vi "HumanDashRead.vi"() -> (1 "DriveMode":T1, 2 "SlowMode":bool, 3 "FieldOriented":bool)   [LabVIEW 2023]
doc: "Human Network\n\nInput\n --Error in \n\nOutput\n --Error out"
uses:
  HumanGlobal.vi
  <vilib>/Rock Robotics/Network Tables/NT Read Boolean.vi
  <vilib>/Rock Robotics/Network Tables/NT Read Number.vi
  HumanDriveModeENUM.ctl
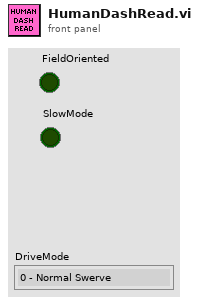
[diagram p1: front panel]
types:
  T1 = typedef "HumanDriveModeENUM.ctl" = enum16{"0 - Normal Swerve", "1 - Auto traj  - Left Speaker", "2 - Auto traj - Center Speaker", "3 - Auto traj - Speaker Right", "4 - Auto traj - Amp", "5 - Auto traj - Source", "6 - Auto traj -  Left Stage", "7 - Auto traj - Center Stage", "8 - Auto traj - Right Stage"}
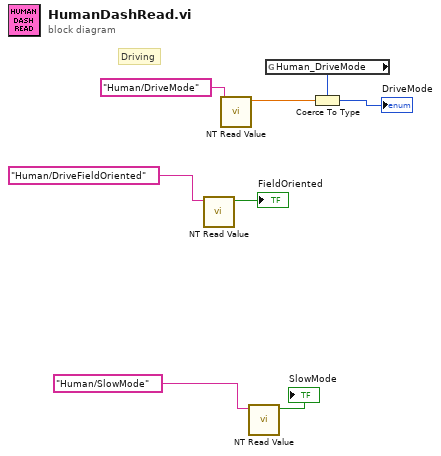
[diagram p0: block diagram]
diagram:
  # "Driving"
  n1 = call-poly <vilib>:"NT Read Value.vi"("name"="Human/DriveFieldOriented") -> ("value"=→"FieldOriented":bool)  [unwired: 8 in, 2 out]
  n2 = call-poly <vilib>:"NT Read Value.vi"("name"="Human/DriveMode") -> ("value"=w3:dbl)  [unwired: 8 in, 2 out]
  n3 = call-poly <vilib>:"NT Read Value.vi"("name"="Human/SlowMode") -> ("value"=→"SlowMode":bool)  [unwired: 8 in, 2 out]
  n4 = global read "HumanGlobal.vi" "Human_DriveMode"() -> (w2:T1)
  n5 = Coerce To Type(0:w3, 1:w2) -> (2:→"DriveMode":T1)
